vi "Standard Bus LUT INI File Path--Constant.vi"() -> (0 "Standard Bus Register LUT Path":path=path "C:/Repos/thermal-chamber-module/Libraries/Thermal Chamber/Documentation/Standard Bus Register Table.ini")   [LabVIEW 2024, in "Watlow F4T.lvclass"]
uses:
  Watlow F4T.lvclass
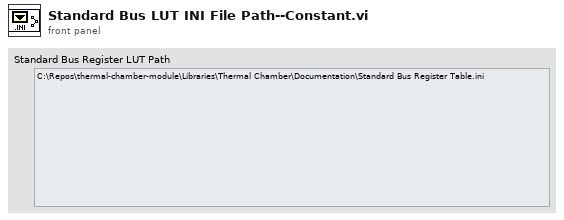
[diagram p1: front panel]
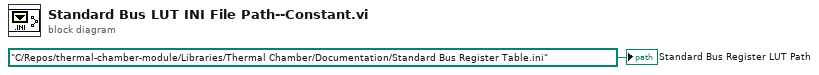
[diagram p0: block diagram]
diagram:
  "Standard Bus Register LUT Path" <- path "C:/Repos/thermal-chamber-module/Libraries/Thermal Chamber/Documentation/Standard Bus Register Table.ini" ("Standard Bus Register Look Up Table Path")
